vi "Dialog_Box.vi"(1 "提示信息":string) -> (0 "选择结果":bool)   [LabVIEW 2020]
doc: "Dialog Box.vi是用于Dialog Box Demo.vi的自定义弹出式双按钮对话框。选择“文件>>VI属性>>窗口外观>>自定义”，可查看下列选项：\n调用时显示前面板\n如之前未打开则在运行后关闭\n窗口动作>>模态\n选择“文件>>VI属性>>窗口运行时位置”，可查看下列选项：\n位置>>居中"
panel:
  in  "否":bool caption="取消"
  in  "是":bool caption="确定"
  out "信息显示":string caption="提示"
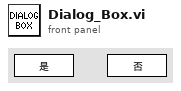
[diagram p1: front panel]
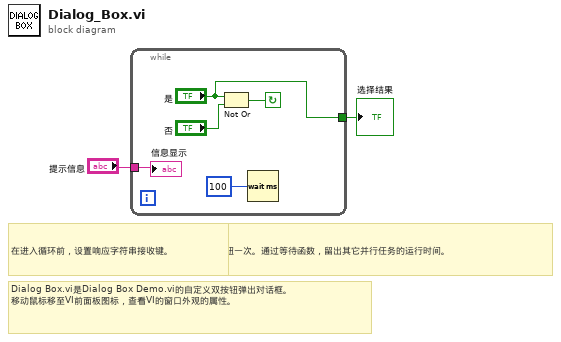
[diagram p0: block diagram]
diagram:
  # "每间隔1/10秒轮询按钮一次。通过等待函数，留出其它并行任务的运行时间。"
  # "Dialog Box.vi是Dialog Box Demo.vi的自定义双按钮弹出对话框。\n移动鼠标移至VI前面板图标，查看VI的窗口外观的属性。"
  # "在进入循环前，设置响应字符串接收键。"
  n1 = while {
    tunnel: ["是"] -> w2
    tunnel: "提示信息" -> [w4]
    stop <- w7 continue-if-true
    n2 = Not Or(1:"否", 2:"是") -> (0:w7:bool)
    n3 = Wait (ms)(milliseconds to wait=u32 100) -> ()  [unwired: 1 out]
    "信息显示" <- w4
  }
  "选择结果" <- w2
